vi "7.-Estructura While y Shift Register.vi"() -> ()   [LabVIEW 2020]
panel:
  out "Waveform Chart":cluster{dbl, "señal":dbl}(graph)
  in  "stop":bool
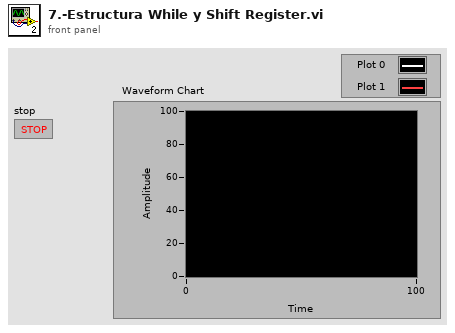
[diagram p1: front panel]
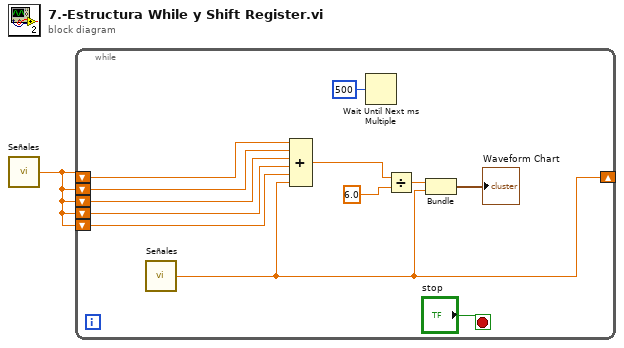
[diagram p0: block diagram]
diagram:
  n1 = call "Señales.vi"() -> ("Señal"=w1:dbl)
  n2 = while {
    shift-right: [w5] -> _
    shift-left: w1 -> [w12]
    shift-left: w1 -> [w11]
    shift-left: w1 -> [w10]
    shift-left: w1 -> [w9]
    shift-left: w1 -> [w8]
    stop <- "stop" stop-if-true
    n3 = call "Señales.vi"() -> ("Señal"=w5:dbl)
    n4 = Compound Arithmetic op=ADD(w12, w11, w10, w9, w8, w5) -> (w13:dbl)
    n5 = Wait Until Next ms Multiple(millisecond multiple=u32 500) -> ()  [unwired: 1 out]
    n6 = Divide(x=w13, y=6.0) -> (x/y=w6:dbl)
    n7 = Bundle "Bundle"(w6, "Señal"=w5) -> (→"Waveform Chart":cluster{dbl, "Señal":dbl})  [unwired: 1 in]
  }
